vi "Raster.vi"(10 "Triangles Sorted":T2[](array[typedef]), 11 "Core Data in":T1) -> (2 "Core Data out":T1, 3 "Delta Time [s]":dbl format="%.3p")   [LabVIEW 2022 SP3]
uses:
  Libraries/3D/3D.lvlib
  90a90ea2-0c49-4de8-9899-23c82480ba68.vi
  46bfe3ef-eb81-4e2a-9a72-195f350e258b.vi
  Scene/Scene.lvclass
  Core Data.ctl
  Application.lvlib
  Libraries/3D/Point 2D.ctl
  Libraries/3D/Triangle 2D.ctl
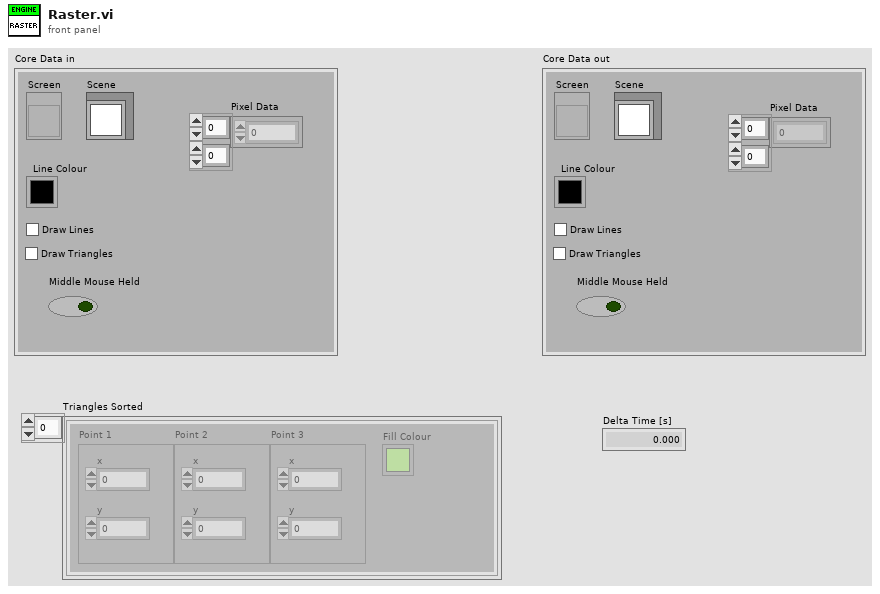
[diagram p1: front panel]
types:
  T1 = typedef "Application.lvlib/Core Data.ctl" = cluster{"Line Colour":u32, "Draw Lines":bool, "Draw Triangles":bool, "Pixel Data":u32[][], "Middle Mouse Held":bool, "Scene":refnum<class "Scene.lvclass">, "Screen":refnum<vi>}
  T2 = typedef "3D.lvlib/Triangle 2D.ctl" = cluster{"Point 1":T3, "Point 2":T3, "Point 3":T3, "Fill Colour":u32}
  T3 = typedef "3D.lvlib/Point 2D.ctl" = cluster{"x":sgl, "y":sgl}
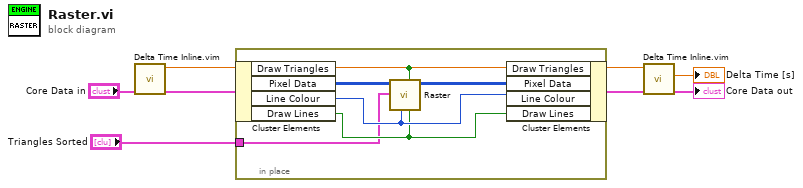
[diagram p0: block diagram]
diagram:
  n1 = call "Delta Time Inline.vim"("value in"="Core Data in") -> ("value out"=w7:T1, "Relative Seconds out [s]"=w5:dbl)  [unwired: 8 in, 1 out]
  n2 = in-place {
    in-place-border: "Triangles Sorted" -> [w8]
    n3 = in-place-cluster #1(w7) -> ("Draw Triangles"=w11:bool, "Pixel Data"=w13:u32[][], "Line Colour"=w10:u32, "Draw Lines"=w9:bool)
    n4 = call "Raster.vi"("Draw Lines"=w9, "Draw Triangles"=w11, "Line Colour"=w10, "Triangles Sorted"=w8, "Pixel Data in"=w13) -> ("Pixel Data out"=w12:u32[][])  [unwired: 6 in]
    n5 = in-place-cluster #1("Draw Triangles"=w11, "Pixel Data"=w12, "Line Colour"=w10, "Draw Lines"=w9) -> (w1:T1)
  }
  n6 = call "Delta Time Inline.vim"("value in"=w1, "Relative Seconds in [s]"=w5) -> ("value out"=→"Core Data out":T1, "Delta Time [s]"=→"Delta Time [s]":dbl)  [unwired: 7 in, 1 out]
